vi "set C2 trigger.vi"(8 "error in (no error)":errorcluster, 11 "Waveform in":refnum<class "Waveform.lvclass">) -> (0 "error out":errorcluster, 3 "Waveform out":refnum<class "Waveform.lvclass">)   [LabVIEW 2012, in "Waveform.lvclass"]
uses:
  Waveform.lvclass
  Waveform.lvclass/Waveform.ctl
  <vilib>/DAQmx/configure/timing.llb/DAQmx Timing (Implicit).vi
  <resource>/objmgr/daqmx.rc
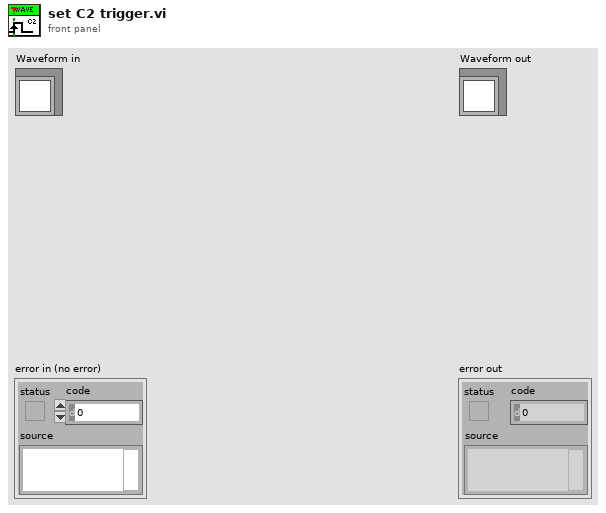
[diagram p1: front panel]
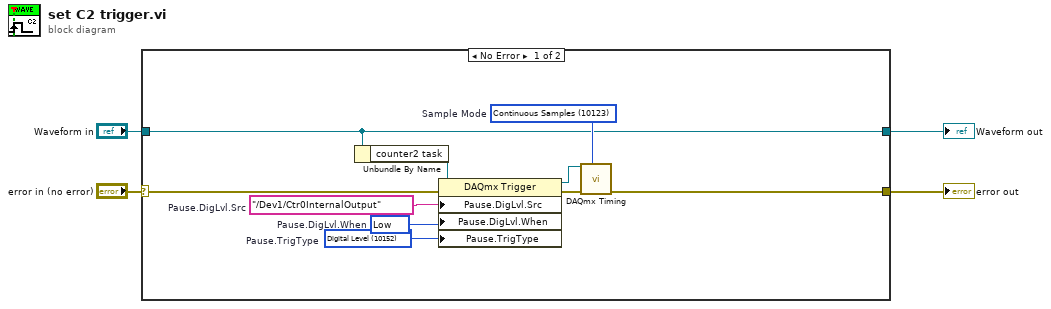
[diagram p0: block diagram]
diagram:
  n1 = case shown="No Error" "error in (no error)" {
    selector: "error in (no error)" -> [w14 w16]
    tunnel: [w5 w16] -> w3
    tunnel: [w7 w15] -> w1
    tunnel: "Waveform in" -> [w7 w15]
    frame No Error {
      w9 = 10123 items=["Finite Samples"=10178, "Continuous Samples"=10123, "Hardware Timed Single Point"=12522]  # Sample Mode
      w11 = 10152 items=["Analog Level"=10101, "Analog Window"=10103, "Digital Level"=10152, "Digital Pattern"=10398, "None"=10230]  # Pause.TrigType
      w12 = 10214 items=["High"=10192, "Low"=10214]  # Pause.DigLvl.When
      w6 = tag "/Dev1/Ctr0InternalOutput"  # Pause.DigLvl.Src
      n2 = Unbundle By Name(w7) -> ("counter2 task"=w13:refnum<k21>)
      n3 = property class="DAQmx Trigger"(reference=w13, error in=w14, "Pause.DigLvl.Src"=w6, "Pause.DigLvl.When"=w12, "Pause.TrigType"=w11) -> (reference out=w8:refnum<k21>, error out=w10:errorcluster)
      n4 = call-poly <vilib>:"DAQmx Timing.vi"("task/channels in"=w8, "sample mode"=w9, "error in"=w10) -> ("error out"=w5:errorcluster)  [unwired: 11 in, 1 out]
    }
    frame Error {
    }
  }
  "error out" <- w3
  "Waveform out" <- w1
